vi "Library Open File.vi"(4 "error in (no error)":errorcluster, 5 "deny mode (deny none)":T2(ring)=enum."deny none", 6 "open mode (read/write)":T1(ring), 7 "file path":path) -> (0 "error out":errorcluster, 3 "refnum":refnum<file>)   [LabVIEW 2012]
doc: "This is a drop-in replacement for the LabVIEW \"open file\" node with as only enhancement less useless error reporting through showing the path of the file that could not be opened as part of the error message."
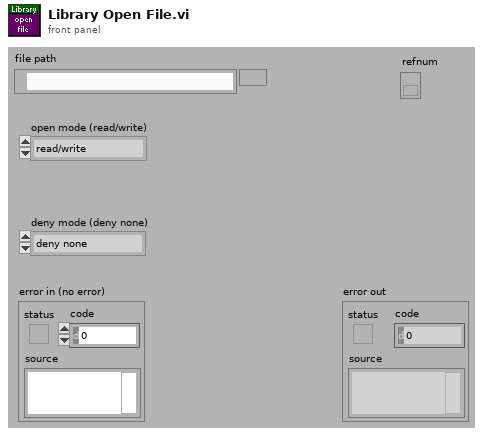
[diagram p1: front panel]
types:
  T1 = enum16{"read/write", "read-only", "write-only", "write-only (truncate)"}
  T2 = enum16{"deny read/write", "deny write-only", "deny none"}
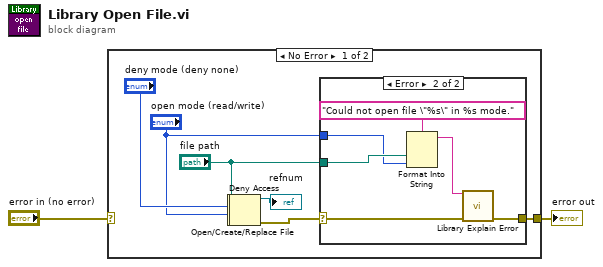
[diagram p0: block diagram]
diagram:
  n1 = case shown="No Error" "error in (no error)" {
    selector: "error in (no error)" -> [_ w18]
    tunnel: [w6 w18] -> w2
    frame No Error {
      n2 = Open/Create/Replace File(file path (use dialog)="file path", access (0:read/write)="open mode (read/write)") -> (refnum out=w3:refnum<file>, error out=w4:errorcluster)  [unwired: 4 in, 1 out]
      n3 = Deny Access(4:w4, 6:"deny mode (deny none)", 7:w3) -> (0:w8:errorcluster, 3:→"refnum":refnum<file>)
      n4 = case shown="Error" w8 {
        selector: w8 -> [w11 w12]
        tunnel: "file path" -> [_ w16]
        tunnel: [w11 w13] -> w6
        tunnel: "open mode (read/write)" -> [_ w15]
        frame No Error {
        }
        frame Error {
          n5 = Format Into String(format string="Could not open file \"%s\" in %s mode.", w16, w15) -> (resulting string=w14:string)  [unwired: 2 in, 1 out]
          n6 = call "Library Explain Error.vi"("explanation prefix (none)"=w14, "error in (no error)"=w12) -> ("explained error"=w13:errorcluster)  [unwired: 13 in]
        }
      }
    }
    frame Error {
    }
  }
  "error out" <- w2
